vi "Copy octprog.vi"(8 "error in":errorcluster, 10 "Destination Path":path, 11 "lvProject path":path) -> (0 "error out":errorcluster)   [LabVIEW 2013]
doc: "This VI copies \"/octprog\" folder to build folder skipping hidden files. This is used to leave out auxiliary local files from the build without need to update project files list everytime something is changed in the octprog folder."
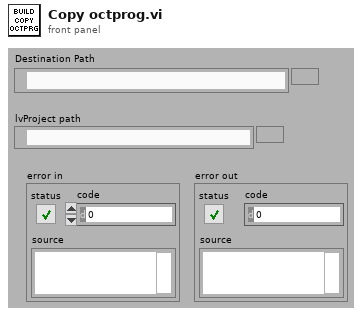
[diagram p1: front panel]
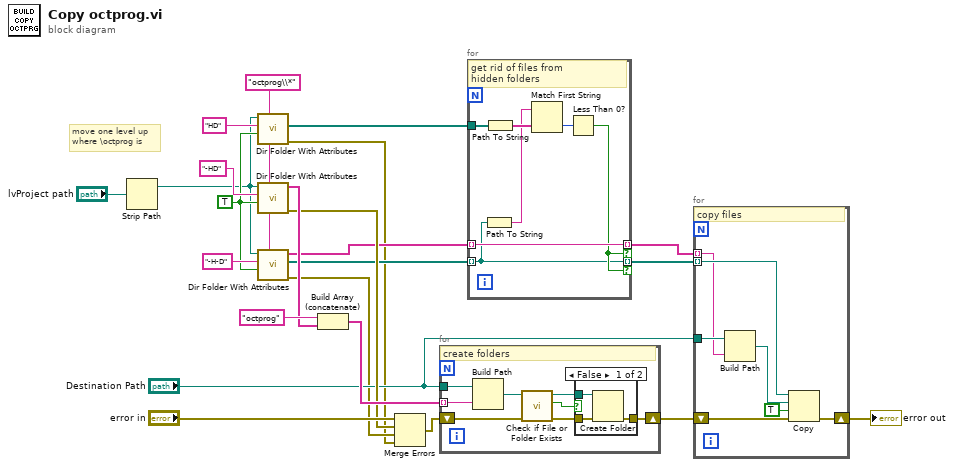
[diagram p0: block diagram]
diagram:
  w11 = TRUE ("recoursive subfolders (/S)? (false)")
  w10 = "octprog\\*" ("wildcard serach key (*)")
  # "move one level up\nwhere \\octprog is"
  n1 = Strip Path(path="lvProject path") -> (stripped path=w1:path)  [unwired: 1 out]
  n2 = call "Dir Folder With Attributes.vi"("wildcard serach key (*)"=w10, "recoursive subfolders (/S)? (false)"=w11, "\"DIR /A:?\" attribute(s) (default: -H)"="HD" ("\"DIR /A:?\" attribute(s) (default: -H)"), "folder"=w1) -> ("error out"=w2:errorcluster, "file/folder paths"=w8:path[])  [unwired: 5 in, 1 out]
  n3 = call "Dir Folder With Attributes.vi"("wildcard serach key (*)"=w10, "recoursive subfolders (/S)? (false)"=w11, "\"DIR /A:?\" attribute(s) (default: -H)"="-HD" ("\"DIR /A:?\" attribute(s) (default: -H)"), "folder"=w1) -> ("error out"=w16:errorcluster, "file/folder names"=w21:string[])  [unwired: 5 in, 1 out]
  n4 = call "Dir Folder With Attributes.vi"("wildcard serach key (*)"=w10, "recoursive subfolders (/S)? (false)"=w11, "\"DIR /A:?\" attribute(s) (default: -H)"="-H-D" ("\"DIR /A:?\" attribute(s) (default: -H)"), "folder"=w1) -> ("error out"=w3:errorcluster, "file/folder paths"=w6:path[], "file/folder names"=w7:string[])  [unwired: 5 in]
  n5 = Build Array (concatenate)("octprog" ("\"DIR /A:?\" attribute(s) (default: -H)"), w21) -> (w20:string[])
  n6 = Merge Errors("error in", w16, w3, w2) -> (w18:errorcluster)
  n7 = for {
    shift-right: [w31] -> w15
    shift-left: w18 -> [w28]
    tunnel: "Destination Path" -> [w30]
    tunnel: w20 -> [w29] mode=indexing
    # "create folders"
    n8 = Build Path(base path=w30, name or relative path=w29) -> (appended path=w27:path)
    n9 = call <vilib>:"Check if File or Folder Exists.vi"("error in (no error)"=w28, "path"=w27) -> ("error out"=w26:errorcluster, "file or folder exists?"=w24:bool, "dup path"=w25:path)  [unwired: 7 in]
    n10 = case shown="False" w24 {
      tunnel: w26 -> [w34 w35]
      tunnel: [w33 w35] -> w31
      tunnel: w25 -> [w32 _]
      frame False {
        n11 = Create Folder(path (use dialog)=w32, error in=w34) -> (error out=w33:errorcluster)  [unwired: 1 in, 2 out]
      }
      frame True {
      }
    }
  }
  n12 = for {
    tunnel: w8 -> [w42]
    tunnel: [w40] -> w4 mode=indexing if=w38
    tunnel: w7 -> [w40] mode=indexing
    tunnel: w6 -> [w37] mode=indexing
    tunnel: [w37] -> w5 mode=indexing if=w38
    # "get rid of files from\nhidden folders"
    n13 = Path To String(path=w37) -> (string=w36:string)
    n14 = Path To String(path=w42) -> (string=w41:string[])
    n15 = Match First String(2:w41, 3:w36) -> (0:w39:i32)  [unwired: 1 out]
    n16 = Less Than 0?(x=w39) -> (x < 0?=w38:bool)
  }
  n17 = for {
    shift-right: [w48] -> w13
    shift-left: w15 -> [w49]
    tunnel: w5 -> [w47] mode=indexing
    tunnel: "Destination Path" -> [w46]
    tunnel: w4 -> [w45] mode=indexing
    # "copy files"
    n18 = Build Path(base path=w46, name or relative path=w45) -> (appended path=w44:path)
    n19 = Copy(8:w49, 9:TRUE ("overwrite (F)"), 10:w44, 11:w47) -> (0:w48:errorcluster)  [unwired: 1 in, 2 out]
  }
  "error out" <- w13
